vi "Tree_Setup for dialog.vi"(7 "Action":T1, 8 "error in":errorcluster, 11 "Tree Ref":refnum<vi>[](array[refnum])) -> (0 "error out":errorcluster, 3 "Tree Ref Out":refnum<vi>[](array[refnum]))   [LabVIEW 2023]
doc: "This VI sets up tree-level, but NOT row-level settings.\n\nDoes not set tree value."
uses:
  controls/action enum.ctl
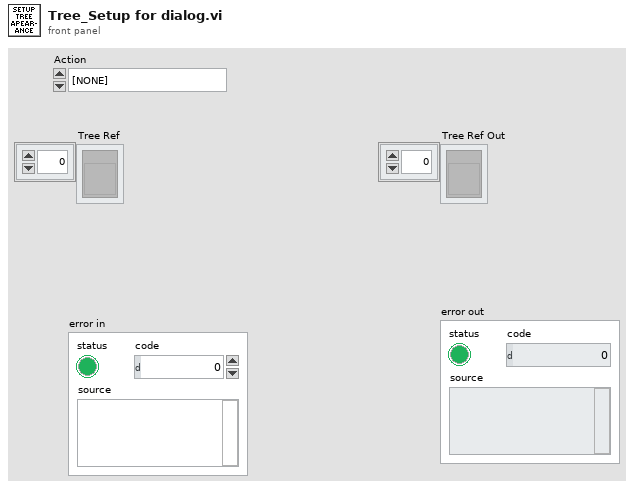
[diagram p1: front panel]
types:
  T1 = typedef "action enum.ctl" = enum16{"[NONE]", "APP_SEPARATOR", "Wire Bundle", "Wire Unbundle", "Terminal Unbundle", "Terminal Bundle", "Bundler Move Up", "Bundler Move Down", "Bundler Insert", "Bundler Remove", "Bundler Remove Unwired", "Bundler Rearrange", "In Place Insert", "In Place Remove", "In Place Remove Unwired", "In Place Rearrange", "Wire Properties", "Wire Method", "Terminal Properties", "Terminal Method", "Property Move Up", "Property Move Down", "Properties Insert", "Properties Remove", "Properties Remove Unwired", "Properties Rearrange", "Method Change", "Class For Constant", "Class For Control", "Class For Node", "Class Name to Clipboard"}
  T2 = enum16{"[NONE]", "Wire Bundle", "Wire Unbundle", "Terminal Unbundle", "Terminal Bundle", "Bundler Insert", "Bundler Remove", "Bundler Remove Unwired", "Bundler Rearrange", "In Place Insert", "In Place Remove", "In Place Remove Unwired", "In Place Rearrange", "Wire Properties", "Wire Method", "Terminal Properties", "Terminal Method", "Properties Insert", "Properties Remove", "Properties Remove Unwired", "Properties Rearrange", "Method Change", "Class for Constant", "Class For Control", "Class For Node", "Class Name to Clipboard"}
  T3 = enum32{"None", "LabVIEW", "Mac OS", "Windows", "Default"}
  T4 = enum8{"Enabled", "Disabled", "Disabled and Grayed Out"}
  T5 = enum16{"None", "Cluster", "Property", "Method", "Class"}
  T6 = cluster{"image type":i32, "image depth":i32, "image":u8[], "mask":u8[], "colors":u32[], "Rectangle":cluster{"left":i16, "top":i16, "right":i16, "bottom":i16}}
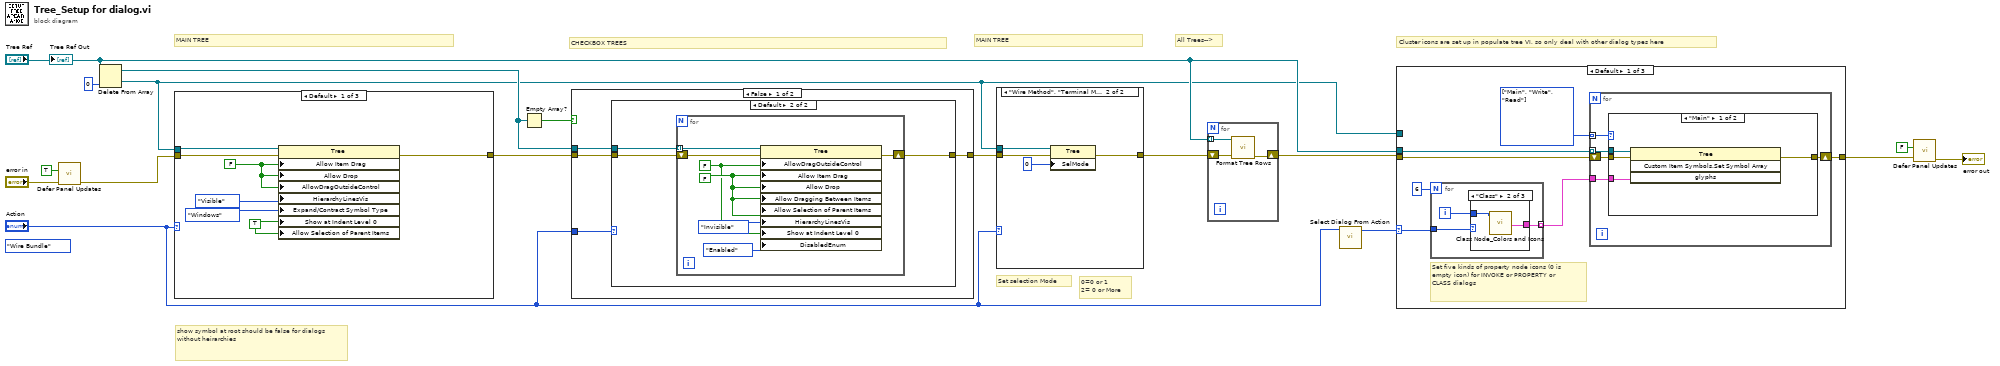
[diagram p0: block diagram]
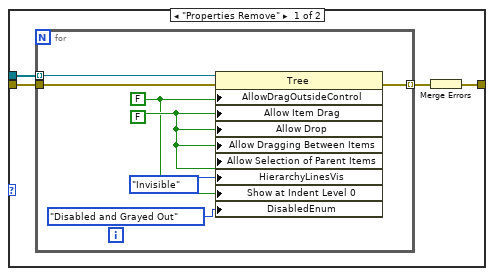
[diagram p2: hidden frame]
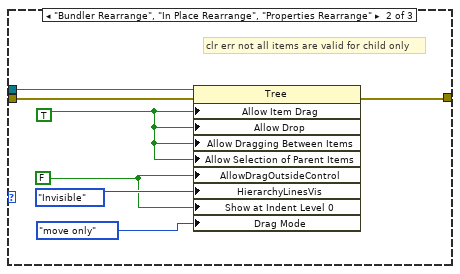
[diagram p4: hidden frame]
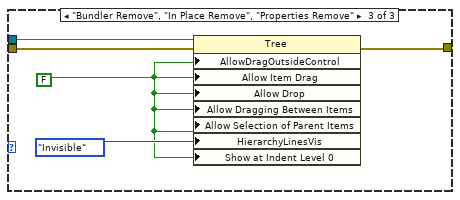
[diagram p5: hidden frame]
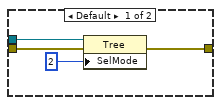
[diagram p6: hidden frame]
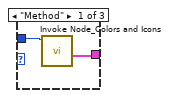
[diagram p7: hidden frame]
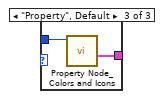
[diagram p8: hidden frame]
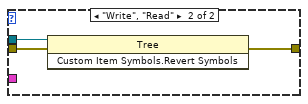
[diagram p9: hidden frame]
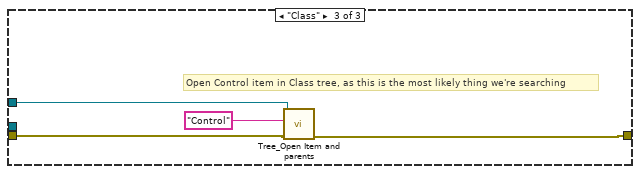
[diagram p11: hidden frame]
diagram:
  (unwired) T2."Wire Bundle" ("Action")
  # "Cluster icons are set up in populate tree VI, so only deal with other dialog types here"
  # "All Trees-->"
  # "MAIN TREE"
  # "show symbol at root should be false for dialogs without heirarchies"
  # "CHECKBOX TREES"
  # "MAIN TREE"
  # "Set selection Mode"
  # "0=0 or 1\n2= 0 or More"
  n1 = call "Defer Panel Updates.vi"("error in (no error)"="error in", "Defer Panel Updates [T]"=TRUE) -> ("error out"=w10:errorcluster)  [unwired: 8 in, 1 out]
  n2 = Delete From Array(array="Tree Ref", index=0) -> (deleted portion=w1:refnum<vi>, array with subset deleted=w4:refnum<vi>[])  [unwired: 1 in]
  n3 = case shown="Default" "Action" {
    tunnel: w1 -> [w24 w31 w36]
    tunnel: [w22 w25 w34] -> w8
    tunnel: w10 -> [w23 w30 w35]
    frame Default {
      w20 = TRUE
      w19 = FALSE
      n4 = property class="Tree"(reference=w24, error in=w23, "Allow Item Drag"=w19, "Allow Drop"=w19, "AllowDragOutsideControl"=w19, "HierarchyLinesVis"=enum32{"Visible", "Invisible", "OS Default"}."Visible" ("Visible Items:Hierarchy Lines Visible"), "Expand/Contract Symbol Type"=T3."Windows" ("Expand/Contract Symbol:Symbol Type"), "Show at Indent Level 0"=w20, "Allow Selection of Parent Items"=w20) -> (error out=w22:errorcluster)  [unwired: 1 out]
    }
    frame "Bundler Rearrange", "In Place Rearrange", "Properties Rearrange" {
      w26 = TRUE
      w27 = FALSE
      # "clr err not all items are valid for child only"
      n5 = property class="Tree"(reference=w31, error in=w30, "Allow Item Drag"=w26, "Allow Drop"=w26, "Allow Dragging Between Items"=w26, "Allow Selection of Parent Items"=w26, "AllowDragOutsideControl"=w27, "HierarchyLinesVis"=enum32{"Visible", "Invisible", "OS Default"}."Invisible" ("Visible Items:Hierarchy Lines Visible"), "Show at Indent Level 0"=w27, "Drag Mode"=enum32{"copy or move", "copy only", "move only"}."move only" ("Drag/Drop:Drag Mode")) -> (error out=w25:errorcluster)  [unwired: 1 out]
    }
    frame "Bundler Remove", "In Place Remove", "Properties Remove" {
      w32 = FALSE
      n6 = property class="Tree"(reference=w36, error in=w35, "AllowDragOutsideControl"=w32, "Allow Item Drag"=w32, "Allow Drop"=w32, "Allow Dragging Between Items"=w32, "Allow Selection of Parent Items"=w32, "HierarchyLinesVis"=enum32{"Visible", "Invisible", "OS Default"}."Invisible" ("Visible Items:Hierarchy Lines Visible"), "Show at Indent Level 0"=w32) -> (error out=w34:errorcluster)  [unwired: 1 out]
    }
  }
  n7 = Empty Array?(array=w4) -> (empty?=w5:bool)
  n8 = case shown="False" w5 {
    tunnel: w4 -> [w40 _]
    tunnel: w8 -> [w39 w62]
    tunnel: [w38 w62] -> w7
    tunnel: "Action" -> [w37 _]
    frame False {
      n9 = case shown="Default" w37 {
        tunnel: w40 -> [w44 w54]
        tunnel: w39 -> [w43 w53]
        tunnel: [w41 w52] -> w38
        frame "Properties Remove" {
          n10 = for {
            tunnel: w44 -> [w51] mode=indexing
            tunnel: w43 -> [w50]
            tunnel: [w49] -> w42 mode=indexing
            w47 = FALSE
            w46 = FALSE
            n11 = property class="Tree"(reference=w51, error in=w50, "AllowDragOutsideControl"=w46, "Allow Item Drag"=w47, "Allow Drop"=w47, "Allow Dragging Between Items"=w47, "Allow Selection of Parent Items"=w47, "HierarchyLinesVis"=enum32{"Visible", "Invisible", "OS Default"}."Invisible" ("Visible Items:Hierarchy Lines Visible"), "Show at Indent Level 0"=w46, "DisabledEnum"=T4."Disabled and Grayed Out" ("Disabled")) -> (error out=w49:errorcluster)  [unwired: 1 out]
          }
          n12 = Merge Errors(w42) -> (w41:errorcluster)
        }
        frame Default {
          n13 = for {
            tunnel: w54 -> [w61] mode=indexing
            shift-right: [w59] -> w52
            shift-left: w53 -> [w60]
            w57 = FALSE
            w56 = FALSE
            n14 = property class="Tree"(reference=w61, error in=w60, "AllowDragOutsideControl"=w56, "Allow Item Drag"=w57, "Allow Drop"=w57, "Allow Dragging Between Items"=w57, "Allow Selection of Parent Items"=w57, "HierarchyLinesVis"=enum32{"Visible", "Invisible", "OS Default"}."Invisible" ("Visible Items:Hierarchy Lines Visible"), "Show at Indent Level 0"=w56, "DisabledEnum"=T4."Enabled" ("Disabled")) -> (error out=w59:errorcluster)  [unwired: 1 out]
          }
        }
      }
    }
    frame True {
    }
  }
  n15 = case shown="\"Wire Method\", \"Terminal Method\", \"Class For Constant\"..\"Class For Node\"" "Action" {
    tunnel: w1 -> [w65 w69]
    tunnel: w7 -> [w64 w68]
    tunnel: [w63 w67] -> w17
    frame Default {
      n16 = property class="Tree"(reference=w65, error in=w64, "SelMode"=2 ("Selection Mode")) -> (error out=w63:errorcluster)  [unwired: 1 out]
    }
    frame "Wire Method", "Terminal Method", "Class For Constant".."Class For Node" {
      n17 = property class="Tree"(reference=w69, error in=w68, "SelMode"=0 ("Selection Mode")) -> (error out=w67:errorcluster)  [unwired: 1 out]
    }
  }
  n18 = for {
    tunnel: "Tree Ref" -> [w71] mode=indexing
    shift-right: [w72] -> w16
    shift-left: w17 -> [w73]
    n19 = call "Format Tree Rows.vi"("error in"=w73, "Tree Ref"=w71) -> ("error out"=w72:errorcluster)  [unwired: 8 in, 1 out]
  }
  n20 = call "Select Dialog From Action.vi"("Action"="Action") -> ("Dialog Selection"=w2:T5)  [unwired: 10 in]
  n21 = case shown="Default" w2 {
    selector: w2 -> [w74 _ _]
    tunnel: w16 -> [w80 w102 w105]
    tunnel: [w79 w102 w104] -> w13
    tunnel: "Tree Ref" -> [w78 _ _]
    tunnel: w1 -> [_ _ w106]
    frame Default {
      w75 = enum16{"Main", "Write", "Read"}[] [enum."Main", enum."Write", enum."Read"] items=["Main", "Write", "Read"] ("Tree Type")
      # "Set five kinds of property node icons (0 is empty icon) for INVOKE or PROPERTY or CLASS dialogs"
      n22 = for {
        N: 6 -> [_]
        tunnel: [w82] -> w77 mode=indexing
        tunnel: w74 -> [w81]
        i -> [w83]
        n23 = case shown="\"Class\"" w81 {
          tunnel: w83 -> [w85 w87 w89]
          tunnel: [w84 w86 w88] -> w82
          frame "Method" {
            n24 = call "Invoke Node_Colors and Icons.vi"("Property Type"=w85) -> ("Icon Pixmap"=w84:T6)  [unwired: 8 in, 2 out]
          }
          frame "Class" {
            n25 = call "Class Node_Colors and Icons.vi"("Property Type"=w87) -> ("Icon Pixmap"=w86:T6)  [unwired: 8 in, 2 out]
          }
          frame "Property", Default {
            n26 = call "Property Node_Colors and Icons.vi"("Property Type"=w89) -> ("Icon Pixmap"=w88:T6)  [unwired: 8 in, 2 out]
          }
        }
      }
      n27 = for {
        tunnel: w77 -> [w94]
        tunnel: w78 -> [w93] mode=indexing
        shift-right: [w91] -> w79
        shift-left: w80 -> [w92]
        tunnel: w75 -> [w90] mode=indexing
        n28 = case shown="\"Main\"" w90 {
          tunnel: [w95 w99] -> w91
          tunnel: w93 -> [w98 w101]
          tunnel: w92 -> [w97 w100]
          tunnel: w94 -> [w96 _]
          frame "Main" {
            n29 = invoke class="Tree" method="Custom Item Symbols.Set Symbol Array"(reference=w98, error in=w97, "glyphs"=w96) -> (error out=w95:errorcluster)  [unwired: 1 in, 3 out]
          }
          frame "Write", "Read" {
            n30 = invoke class="Tree" method="Custom Item Symbols.Revert Symbols"(reference=w101, error in=w100) -> (error out=w99:errorcluster)  [unwired: 1 in, 2 out]
          }
        }
      }
    }
    frame "Cluster" {
    }
    frame "Class" {
      # "Open Control item in Class tree, as this is the most likely thing we're searching"
      n31 = call "Tree_Open Item and parents.vi"("error in (no error)"=w105, "Tag"="Control", "TreeControl in"=w106) -> ("error out"=w104:errorcluster)  [unwired: 8 in]
    }
  }
  n32 = call "Defer Panel Updates.vi"("error in (no error)"=w13, "Defer Panel Updates [T]"=FALSE) -> ("error out"=→"error out":errorcluster)  [unwired: 8 in, 1 out]
  "Tree Ref Out" <- "Tree Ref"
